vi "修改密码.vi"(8 "当前用户信息":T1, 9 "管理人员1+密码":string[][](array[string]), 10 "操作人员0+密码":string[][](array[string]), 11 "密码文件路径":path=path "E:/LabVIEW Data/盾构/default") -> (2 "管理人员1+密码_out":string[][](array[string]), 3 "操作人员0+密码_out":string[][](array[string]))   [LabVIEW 2018]
panel:
  out "string用户名":string
  out "string人员类别":string
  in  "返回":bool
  in  "修改密码":bool
  in  "请输入密码":string
  in  "请输入新密码":string
  in  "请重新输入新密码":string
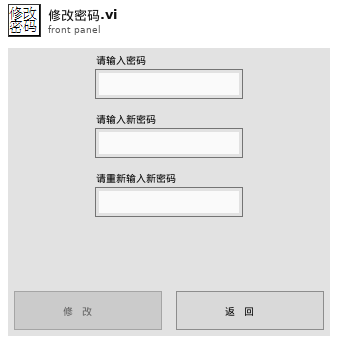
[diagram p1: front panel]
types:
  T1 = cluster{"数值-当前用户类别":u8, "当前用户类别":string, "数值-当前用户名":u16, "当前用户名":string}
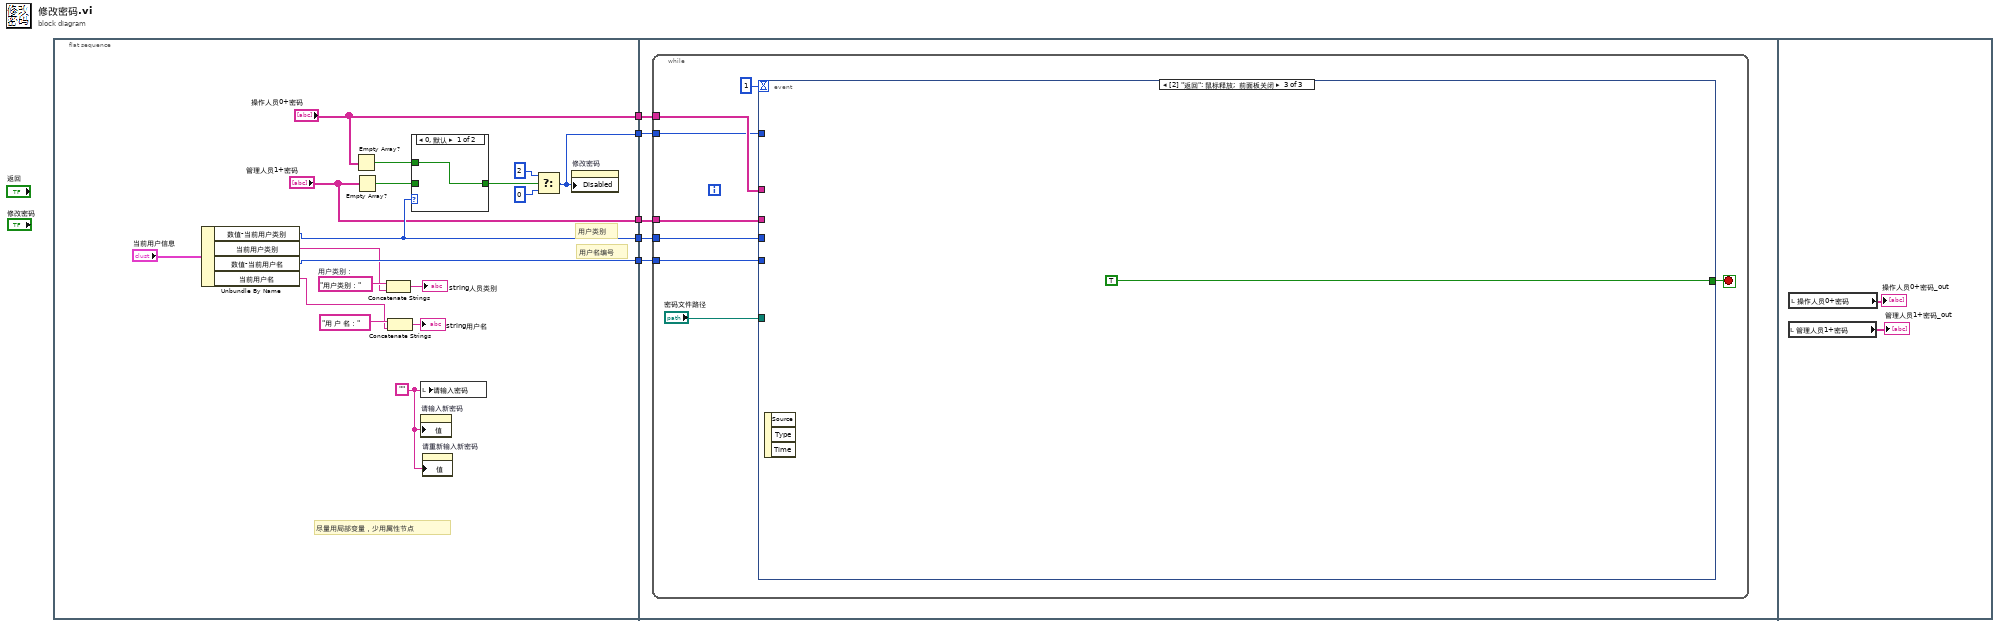
[diagram p0: block diagram]
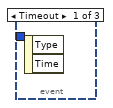
[diagram p3: hidden frame]
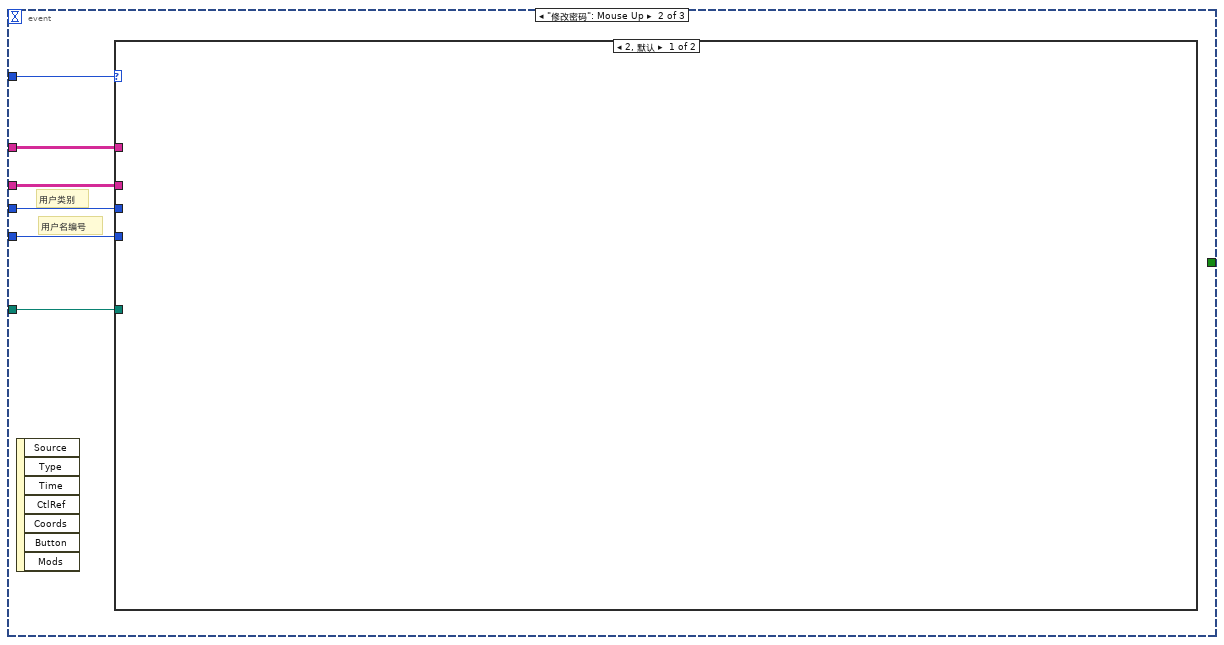
[diagram p4: hidden frame]
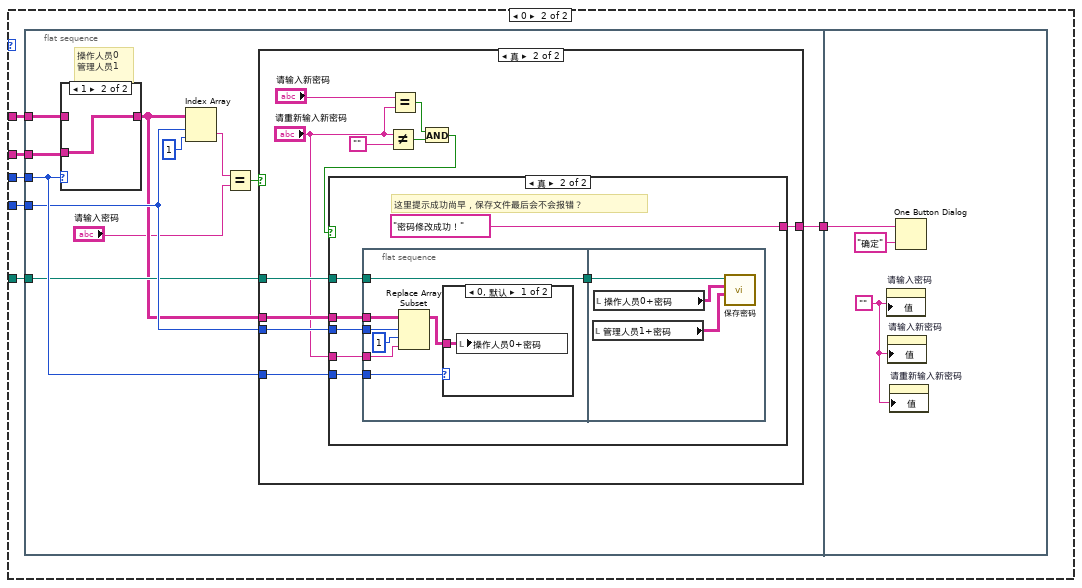
[diagram p5: hidden frame]
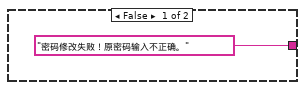
[diagram p6: hidden frame]
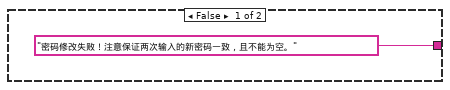
[diagram p7: hidden frame]
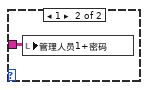
[diagram p8: hidden frame]
diagram:
  n1 = flat-sequence {
    tunnel: [w18] -> w5
    tunnel: [w17] -> w4
    tunnel: ["操作人员0+密码"] -> w3
    tunnel: ["管理人员1+密码"] -> w2
    tunnel: [w7] -> w1
    tunnel: w5 -> [w30]
    tunnel: w4 -> [w29]
    tunnel: w3 -> [w28]
    tunnel: w2 -> [w27]
    tunnel: w1 -> [w26]
    frame #0 {
      w6 = ""
      w23 = "用户类别："  # 用户类别：
      # "尽量用局部变量，少用属性节点"
      # "用户名编号"
      # "用户类别"
      n2 = Unbundle By Name("当前用户信息") -> ("数值-当前用户类别"=w18:u8, "当前用户类别"=w16:string, "数值-当前用户名"=w17:u16, "当前用户名"=w15:string)
      n3 = Empty Array?(array="操作人员0+密码") -> (empty?=w13:bool)
      n4 = Empty Array?(array="管理人员1+密码") -> (empty?=w8:bool)
      n5 = Concatenate Strings(w23, w16) -> (→"string人员类别":string)
      n6 = Concatenate Strings("用 户 名：", w15) -> (→"string用户名":string)
      n7 = case shown="0, 默认" w18 {
        tunnel: w13 -> [w24 _]
        tunnel: [w24 w25] -> w9
        tunnel: w8 -> [_ w25]
        frame 0, Default {
        }
        frame 1 {
        }
      }
      n8 = local write "请输入密码"(w6) -> ()
      n9 = property on="请输入新密码" class="Str"("值"=w6) -> ()  [unwired: 2 in, 2 out]
      n10 = property on="请重新输入新密码" class="Str"("值"=w6) -> ()  [unwired: 2 in, 2 out]
      n11 = Select(t=u8 2 ("禁用"), s=w9, f=u8 0 ("禁用")) -> (s? t:f=w7:u8)
      n12 = property on="修改密码" class="Bool (严格)"("Disabled"=w7) -> ()  [unwired: 2 in, 2 out]
    }
    frame #1 {
      n13 = while {
        tunnel: w30 -> [w36]
        tunnel: w29 -> [w35]
        tunnel: w28 -> [w34]
        tunnel: w27 -> [w33]
        tunnel: w26 -> [w32]
        stop <- w37 stop-if-true
        n14 = event shown="[2] \"返回\": 鼠标释放;  前面板关闭" {
          selector: _ -> [_ _ _]
          dyn-events: _ -> [_ _ _]
          timeout: 1 -> [_ _ _]
          tunnel: w34 -> [_ w43 _]
          tunnel: w33 -> [_ w42 _]
          tunnel: w36 -> [_ w44 _]
          tunnel: w35 -> [_ w41 _]
          tunnel: "密码文件路径" -> [_ w40 _]
          tunnel: [_ _ TRUE] -> w37
          tunnel: w32 -> [_ w39 _]
          event Timeout {
            n15 = event-data() -> ()  [unwired: 1 in, 2 out]
          }
          event "修改密码": Mouse Up {
            # "用户名编号"
            # "用户类别"
            n16 = event-data() -> ()  [unwired: 1 in, 7 out]
            n17 = case shown="2, 默认" w39 {
              tunnel: w44 -> [_ w50]
              tunnel: w43 -> [_ w49]
              tunnel: w42 -> [_ w48]
              tunnel: w41 -> [_ w47]
              tunnel: w40 -> [_ w46]
              frame 2, Default {
              }
              frame 0 {
                n18 = flat-sequence {
                  tunnel: w50 -> [w61]
                  tunnel: w49 -> [w60]
                  tunnel: w48 -> [w59]
                  tunnel: w47 -> [w58]
                  tunnel: w46 -> [w57]
                  tunnel: [w51] -> w45
                  tunnel: w45 -> [w96]
                  frame #0 {
                    # "操作人员0\n管理人员1"
                    n19 = case shown="1" w61 {
                      tunnel: w60 -> [w94 _]
                      tunnel: [w94 w95] -> w54
                      tunnel: w59 -> [_ w95]
                      frame 0, Default {
                      }
                      frame 1 {
                      }
                    }
                    n20 = Index Array(array=w54, index (row)=w58, index (col)=1 ("禁用的索引 (col)")) -> (element=w55:string)
                    n21 = Equal?(x=w55, y="请输入密码") -> (x = y?=w53:bool)
                    n22 = case shown="真" w53 {
                      tunnel: ["密码修改失败！原密码输入不正确。" w69] -> w51
                      tunnel: w54 -> [_ w68]
                      tunnel: w58 -> [_ w67]
                      tunnel: w61 -> [_ w66]
                      tunnel: w57 -> [_ w65]
                      frame False {
                      }
                      frame True {
                        n23 = Not Equal?(x="请重新输入新密码", y="") -> (x != y?=w71:bool)
                        n24 = Equal?(x="请输入新密码", y="请重新输入新密码") -> (x = y?=w72:bool)
                        n25 = And(x=w72, y=w71) -> (x .and. y?=w70:bool)
                        n26 = case shown="真" w70 {
                          tunnel: ["密码修改失败！注意保证两次输入的新密码一致，且不能为空。" "密码修改成功！"] -> w69
                          tunnel: w68 -> [_ w81]
                          tunnel: w67 -> [_ w75]
                          tunnel: "请重新输入新密码" -> [_ w80]
                          tunnel: w66 -> [_ w76]
                          tunnel: w65 -> [_ w79]
                          frame False {
                          }
                          frame True {
                            # "这里提示成功尚早，保存文件最后会不会报错？"
                            n27 = flat-sequence {
                              tunnel: w81 -> [w88]
                              tunnel: w75 -> [w87]
                              tunnel: w80 -> [w85]
                              tunnel: w76 -> [w84]
                              tunnel: w79 -> [w82]
                              tunnel: [w82] -> w78
                              tunnel: w78 -> [w93]
                              frame #0 {
                                n28 = Replace Array Subset(array=w88, new element=w85, index (row)=w87, index (col)=1 ("禁用的索引 (col)")) -> (w83:string[][])
                                n29 = case shown="0, 默认" w84 {
                                tunnel: w83 -> [w89 w90]
                                frame 0, Default {
                                n30 = local write "操作人员0+密码"(w89) -> ()
                                }
                                frame 1 {
                                n31 = local write "管理人员1+密码"(w90) -> ()
                                }
                                }
                              }
                              frame #1 {
                                n32 = local read "管理人员1+密码"() -> (w91:string[][])
                                n33 = local read "操作人员0+密码"() -> (w92:string[][])
                                n34 = call "保存密码.vi"("密码文件路径"=w93, "操作人员0+密码"=w92, "管理人员1+密码"=w91) -> ()  [unwired: 4 in, 1 out]
                              }
                            }
                          }
                        }
                      }
                    }
                  }
                  frame #1 {
                    w98 = ""
                    n35 = property on="请输入密码" class="Str"("值"=w98) -> ()  [unwired: 2 in, 2 out]
                    n36 = property on="请输入新密码" class="Str"("值"=w98) -> ()  [unwired: 2 in, 2 out]
                    n37 = property on="请重新输入新密码" class="Str"("值"=w98) -> ()  [unwired: 2 in, 2 out]
                    n38 = One Button Dialog(message=w96, button name ("OK")="确定" ("按钮名称（“确定”）")) -> ()  [unwired: 1 out]
                  }
                }
              }
            }
          }
          event "返回": Mouse Up; Panel Close {
            n39 = event-data() -> ()  [unwired: 1 in, 3 out]
          }
        }
      }
    }
    frame #2 {
      n40 = local read "管理人员1+密码"() -> (→"管理人员1+密码_out":string[][])
      n41 = local read "操作人员0+密码"() -> (→"操作人员0+密码_out":string[][])
    }
  }
